vi "macro_CreatePathTraj.vi"() -> ()   [LabVIEW 2019, in "PathPlanner24.lvlib"]
uses:
  PathPlanner24.lvlib
  <vilib>/Rock Robotics/WPI/ThirdParty/JAS_Junk/TrajLib/Trajectory_Library.lvlib
  <vilib>/Rock Robotics/WPI/ThirdParty/JAS_Junk/TrajLib/TypeDef/TRANSLATION2D.ctl
  <vilib>/Rock Robotics/WPI/ThirdParty/JAS_Junk/TrajLib/TypeDef/ROTATION2D.ctl
  TypeDef/PathPlannerPathConstraints.ctl
  TypeDef/PathPlannerTrajectoryState.ctl
  TypeDef/PathPlannerTrajectory.ctl
panel:
  out "PathPlannerTrajectory":T1 {"States"."TargetHolonomicRotation"."SIN" format="%13.4f"; "States"."TargetHolonomicRotation"."COS" format="%13.4f"; "States"."TargetHolonomicRotation"."VALUE" format="%13.4f"; "States"."Heading"."SIN" format="%13.4f"; "States"."Heading"."COS" format="%13.4f"; "States"."Heading"."VALUE" format="%13.4f"; "States"."PositionMeters"."Y" format="%14.3f"; "States"."PositionMeters"."X" format="%14.3f"}
  out "Path\nCreation\nError":bool
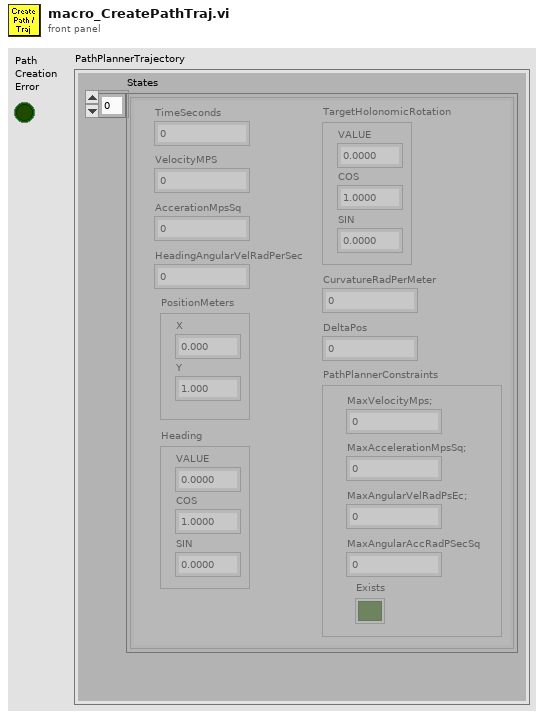
[diagram p1: front panel]
types:
  T1 = typedef "PathPlanner24.lvlib/PathPlannerTrajectory.ctl" = cluster{"States":T2[]}
  T2 = typedef "PathPlanner24.lvlib/PathPlannerTrajectoryState.ctl" = cluster{"TimeSeconds":dbl, "VelocityMPS":dbl, "AccerationMpsSq":dbl, "HeadingAngularVelRadPerSec":dbl, "PositionMeters":T3, "Heading":T4, "TargetHolonomicRotation":T4, "CurvatureRadPerMeter":dbl, "PathPlannerConstraints":T5, "DeltaPos":dbl}
  T3 = typedef "Trajectory_Library.lvlib/TRANSLATION2D.ctl" = cluster{"X":dbl, "Y":dbl}
  T4 = typedef "Trajectory_Library.lvlib/ROTATION2D.ctl" = cluster{"VALUE":dbl, "COS":dbl, "SIN":dbl}
  T5 = typedef "PathPlanner24.lvlib/PathPlannerPathConstraints.ctl" = cluster{"MaxVelocityMps;":dbl, "MaxAccelerationMpsSq;":dbl, "MaxAngularVelRadPsEc;":dbl, "MaxAngularAccRadPSecSq":dbl, "Exists":bool}
  T6 = typedef "Trajectory_Library.lvlib/POSE2D.ctl" = cluster{"TRANSLATION":T3, "ROTATION":T4}
  T7 = typedef "Trajectory_Library.lvlib/CHASSIS_SPEEDS.ctl" = cluster{"vX":dbl, "vY":dbl, "vOmega":dbl}
  T8 = typedef "PathPlanner24.lvlib/PathPlannerGoalEndState.ctl" = cluster{"Velocity":dbl, "Rotation":T4}
  T9 = typedef "PathPlanner24.lvlib/PathPlannerPath.ctl" = cluster{"BezierPoints":T3[], "PreviewStartingRotation":T4, "Reversed":bool, "RotationTargets":T10[], "ConstraintZones":T11[], "EventMarkers":T12[], "GlobalConstraints":T5, "GoalEndState":T8, "AllPoints":T15[]}
  T10 = typedef "PathPlanner24.lvlib/PathPlannerRotationTarget.ctl" = cluster{"target":T4, "WaypointRelativePosition":dbl, "Exists":bool}
  T11 = typedef "PathPlanner24.lvlib/PathPlannerConstraintsZone.ctl" = cluster{"minWaypointPos":dbl, "maxWaypointPos":dbl, "Constraints":T5, "Present":bool}
  T12 = typedef "PathPlanner24.lvlib/PathPlannerEventMarker.ctl" = cluster{"WaypointRelativePos":dbl, "Command":T13}
  T13 = typedef "PathPlanner24.lvlib/PathPlannerCommandUtil.ctl" = cluster{"waitTime":dbl, "name":string, "pathName":string, "commands":cluster{"type":T14, "waitTime":dbl, "name":string, "pathName":string}[], "type":T14}
  T14 = typedef "PathPlanner24.lvlib/PathPlanner_CommandUtilType_ENUM.ctl" = enum16{"Unknown", "Wait", "Named", "Path", "Sequential", "Parallel", "Race", "Deadline"}
  T15 = typedef "PathPlanner24.lvlib/PathPlannerPathPoint.ctl" = cluster{"Position":T3, "HolonomicRotation":T4, "DistAlongPath":dbl, "CurveRadius":dbl, "MaxV":dbl, "Constraints":T5, "HolonomicRotationExists":bool}
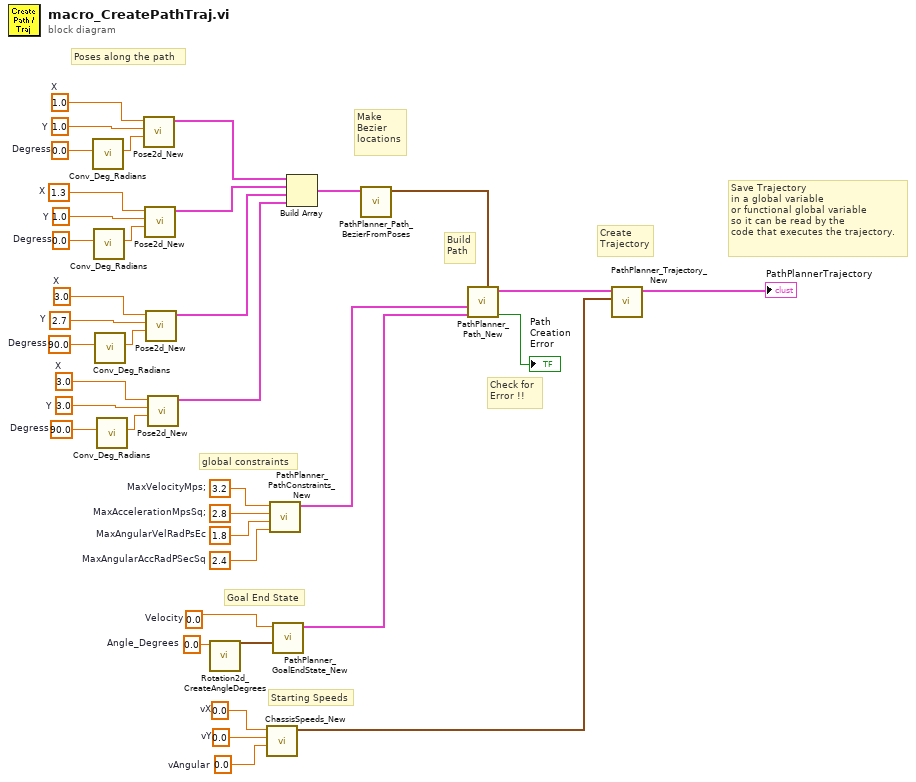
[diagram p0: block diagram]
diagram:
  w2 = 0.0  # vX
  w3 = 0.0  # vY
  w4 = 0.0  # vAngular
  w9 = 0.0  # Angle_Degrees
  w11 = 0.0  # Velocity
  w13 = 3.2  # MaxVelocityMps;
  w14 = 2.8  # MaxAccelerationMpsSq;
  w15 = 1.8  # MaxAngularVelRadPsEc
  w16 = 2.4  # MaxAngularAccRadPSecSq
  w22 = 3.0  # X
  w23 = 3.0  # Y
  w24 = 90.0  # Degress
  w26 = 3.0  # X
  w27 = 2.7  # Y
  w28 = 90.0  # Degress
  w30 = 1.3  # X
  w31 = 1.0  # Y
  w32 = 0.0  # Degress
  w34 = 1.0  # X
  w35 = 1.0  # Y
  w36 = 0.0  # Degress
  # "Save Trajectory\nin a global variable\nor functional global variable\nso it can be read by the \ncode that executes the trajectory."
  # "Create\nTrajectory"
  # "Check for\nError !!"
  # "Starting Speeds"
  # "Goal End State"
  # "global constraints"
  # "Make\nBezier\nlocations"
  # "Build\nPath"
  # "Poses along the path"
  n1 = call <vilib>:"Conv_Deg_Radians.vi"("Degress"=w36) -> ("Radians"=w37:dbl)  [unwired: 10 in]
  n2 = call <vilib>:"Conv_Deg_Radians.vi"("Degress"=w32) -> ("Radians"=w33:dbl)  [unwired: 10 in]
  n3 = call <vilib>:"Conv_Deg_Radians.vi"("Degress"=w28) -> ("Radians"=w29:dbl)  [unwired: 10 in]
  n4 = call <vilib>:"Conv_Deg_Radians.vi"("Degress"=w24) -> ("Radians"=w25:dbl)  [unwired: 10 in]
  n5 = call <vilib>:"Pose2d_New.vi"("Heading"=w37, "Y"=w35, "X"=w34) -> ("out POSe"=w21:T6)  [unwired: 8 in]
  n6 = call <vilib>:"Pose2d_New.vi"("Heading"=w33, "Y"=w31, "X"=w30) -> ("out POSe"=w20:T6)  [unwired: 8 in]
  n7 = call <vilib>:"Pose2d_New.vi"("Heading"=w29, "Y"=w27, "X"=w26) -> ("out POSe"=w19:T6)  [unwired: 8 in]
  n8 = call <vilib>:"Pose2d_New.vi"("Heading"=w25, "Y"=w23, "X"=w22) -> ("out POSe"=w18:T6)  [unwired: 8 in]
  n9 = call <vilib>:"Rotation2d_CreateAngleDegrees.vi"("Angle_Degrees"=w9) -> ("ROTATION"=w10:T4)  [unwired: 10 in]
  n10 = call <vilib>:"ChassisSpeeds_New.vi"("vAngular"=w4, "vY"=w3, "vX"=w2) -> ("CHASSIS"=w1:T7)  [unwired: 8 in]
  n11 = call "PathPlanner_PathConstraints_New.vi"("MaxAngularAccRadPSecSq"=w16, "MaxAngularVelRadPsEc;"=w15, "MaxAccelerationMpsSq;"=w14, "MaxVelocityMps;"=w13) -> ("PathPlannerConstraints"=w12:T5)  [unwired: 7 in]
  n12 = call "PathPlanner_GoalEndState_New.vi"("Rotation"=w10, "Velocity"=w11) -> ("GoalEndState"=w8:T8)  [unwired: 9 in]
  n13 = Build Array(w21, w20, w19, w18) -> (w38:T6[])
  n14 = call "PathPlanner_Path_BezierFromPoses.vi"("Poses"=w38) -> ("Bezier"=w17:T3[])  [unwired: 9 in, 1 out]
  n15 = call "PathPlanner_Path_New.vi"("BezierPoints"=w17, "GoalEndState"=w8, "GlobalConstraints"=w12) -> ("Error"=→"Path\nCreation\nError":bool, "PathPlannerPath"=w6:T9)  [unwired: 7 in]
  n16 = call "PathPlanner_Trajectory_New.vi"("StartingSpeeds"=w1, "Path"=w6) -> ("PathPlannerTrajectory"=→"PathPlannerTrajectory":T1)  [unwired: 8 in, 1 out]
